vi "Run_Core.vi"(0 "Message Popup in":refnum<class "Arithmetic Operations.lvclass">, 11 "error in (no error)":errorcluster) -> (4 "Message Popup out":refnum<class "Arithmetic Operations.lvclass">, 6 "Return":variant, 15 "error out":errorcluster)   [LabVIEW 2016, in "Arithmetic Operations.lvclass"]
uses:
  Arithmetic Operations.lvclass
  D:/TOOLS/LabVIEW-Script-Language.git/trunk/source code/LSL components/functions/functionsbase/functionbase.lvclass
  functionsbase/functionbase.lvclass/functionbase.ctl
  Arithmetic Operations.lvclass/Arithmetic Operations.ctl
  functionsbase/properties/Read Smart Syntax Representation.vi
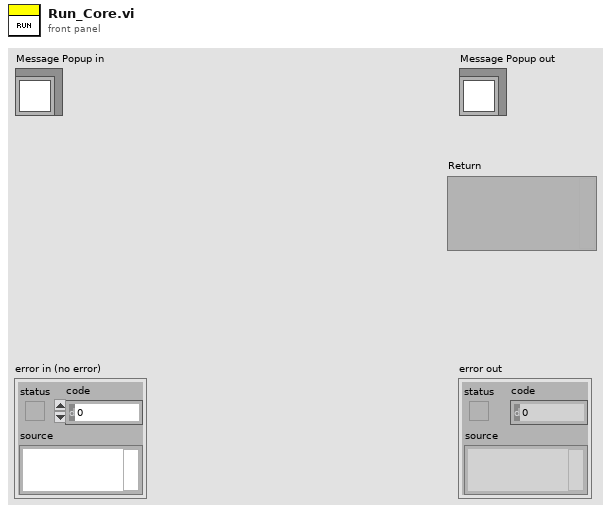
[diagram p1: front panel]
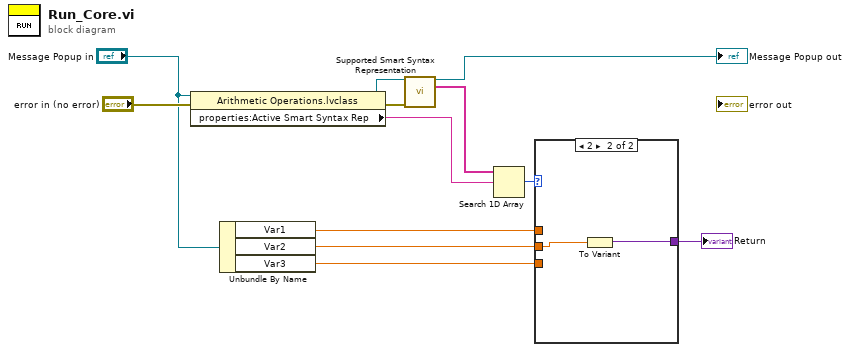
[diagram p0: block diagram]
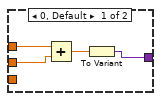
[diagram p2: hidden frame]
diagram:
  n1 = property class="Arithmetic Operations.lvclass"(reference="Message Popup in", error in="error in (no error)") -> (reference out=w8:refnum<class "Arithmetic Operations.lvclass">, error out=w11:errorcluster, "properties:Active Smart Syntax Rep"=w5:string)
  n2 = Unbundle By Name("Message Popup in") -> ("Var1"=w4:dbl, "Var2"=w3:dbl, "Var3"=w2:dbl)
  n3 = call-dynamic "Supported Smart Syntax Representation.vi"("Message Popup in"=w8, "error in (no error)"=w11) -> ("Message Popup out"=→"Message Popup out":refnum<class "Arithmetic Operations.lvclass">, "Smart Syntax Representation List"=w10:string[])  [unwired: 11 in, 1 out]
  n4 = Search 1D Array(1D array=w10, element=w5) -> (index of element=w9:i32)  [unwired: 1 in]
  n5 = case shown="2" w9 {
    tunnel: w4 -> [w16 _]
    tunnel: w3 -> [w15 w18]
    tunnel: w2 -> [_ _]
    tunnel: [w13 w17] -> w1
    frame 0, Default {
      n6 = Add(x=w16, y=w15) -> (x+y=w14:dbl)
      n7 = To Variant(anything=w14) -> (Variant=w13:variant)
    }
    frame 2 {
      n8 = To Variant(anything=w18) -> (Variant=w17:variant)
    }
  }
  "Return" <- w1
